vi "FunctionalResistanceGlobal.vi"(7 "FUNCTION":enum16{"SET RESISTANCE", "READ RESISTANCE"}(ring), 10 "RESISTANCE IN":sgl format="%^_6e") -> (2 "RESISTANCE OUT":sgl format="%^_6e")   [LabVIEW 2012]
doc: "Application example"
panel:
  # "FunctionalResistanceGlobal.vi"
  # "Example on a simple functional global that could be used\nfor transferring resistance into another LabView application.\n\nWriting to the global takes place when function is \"set resistance\"\nand the input is connected to the resistance output of the \nReadAvs47b.vi.  When reading, function is set to \"read resistance\nand input can be left unconnected."
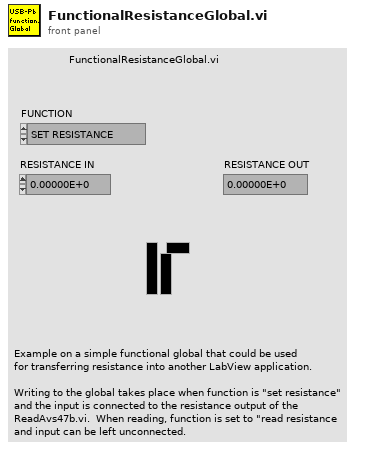
[diagram p1: front panel]
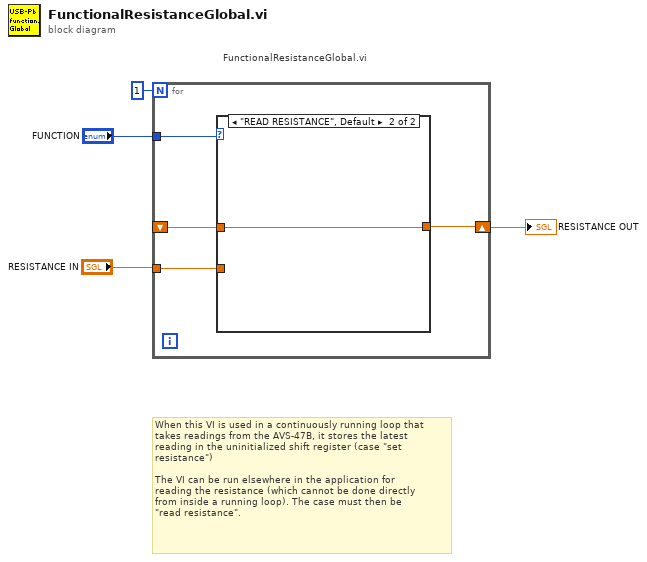
[diagram p0: block diagram]
diagram:
  # "When this VI is used in a continuously running loop that\ntakes readings from the AVS-47B, it stores the latest \nreading in the uninitialized shift register (case \"set\nresistance\")\n\nThe VI can be run elsewhere in the application for \nreading the resistance (which cannot be done directly\nfrom inside a running loop). The case must then be\n\"read resistance\"."
  # "FunctionalResistanceGlobal.vi"
  n1 = for {
    N: 1 -> [_]
    tunnel: "FUNCTION" -> [w8]
    shift-right: [w6] -> w1
    shift-left: _ -> [w5]
    tunnel: "RESISTANCE IN" -> [w7]
    n2 = case shown="\"READ RESISTANCE\", Default" w8 {
      tunnel: w7 -> [w9 _]
      tunnel: [w9 w10] -> w6
      tunnel: w5 -> [_ w10]
      frame "SET RESISTANCE" {
      }
      frame "READ RESISTANCE", Default {
      }
    }
  }
  "RESISTANCE OUT" <- w1
